vi "Inverse_Kinematics.vi"(4 "arm2 length (mm)":dbl, 6 "arm1 length (mm)":dbl, 9 "arm direction":bool, 10 "y (mm)":dbl, 11 "x (mm)":dbl) -> (2 "th2":dbl, 3 "th1":dbl)   [LabVIEW 2017, in "myPAM.lvlib"]
uses:
  myPAM.lvlib
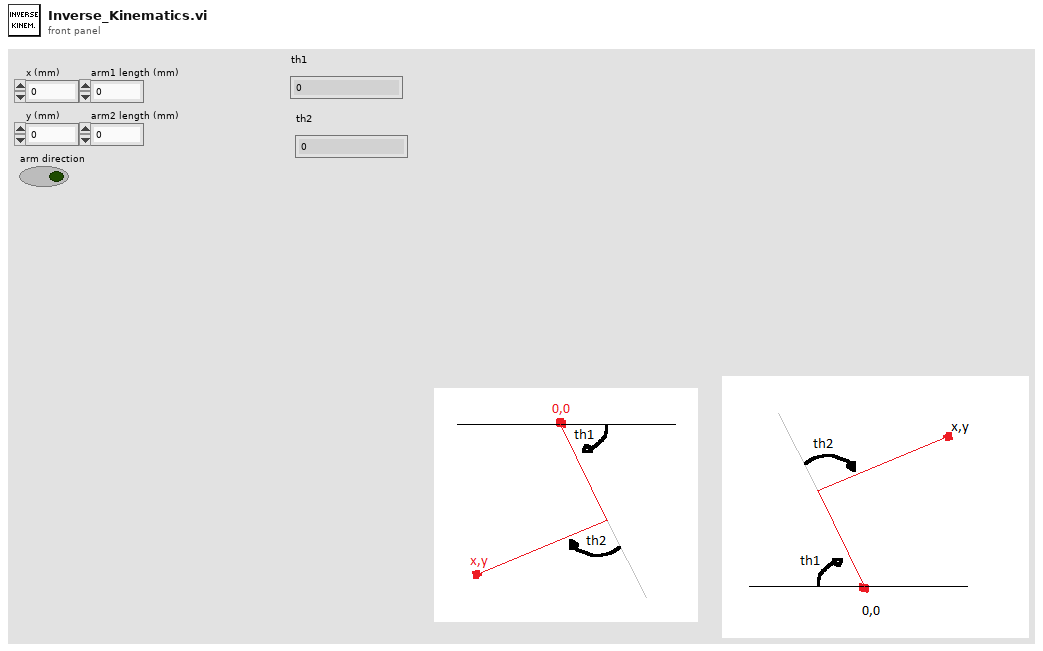
[diagram p1: front panel]
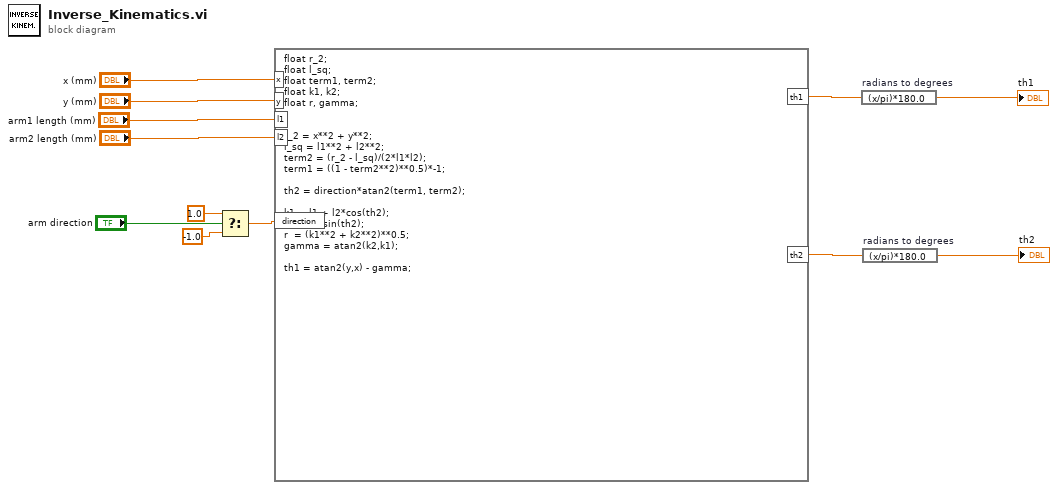
[diagram p0: block diagram]
diagram:
  n1 = Select(t=1.0, s="arm direction", f=-1.0 ("t")) -> (s? t:f=w1:dbl)
  n2 = formula code="float r_2;\nfloat l_sq;\nfloat term1, term2;\nfloat k1, k2;\nfloat r, gamma;\n\n\nr_2 = x**2 + y**2;\nl_sq = l1**2 + l2**2;\nterm2 = (r_2 - l_sq)/(2*l1*l2);\nterm1 = ((1 - term2**2)**0.5)*-1;\n\nth2 = direction*atan2(term1, term2);\n\nk1 = l1 + l2*cos(th2);\nk2 = l2*sin(th2);\nr  = (k1**2 + k2**2)**0.5;\ngamma = atan2(k2,k1);\n\nth1 = atan2(y,x) - gamma;"("x"="x (mm)", "y"="y (mm)", "l1"="arm1 length (mm)", "l2"="arm2 length (mm)", "direction"=w1) -> ("th1"=w4:dbl, "th2"=w5:dbl)
  n3 = expression code="(x/pi)*180.0" "radians to degrees"(w4) -> (→"th1":dbl)
  n4 = expression code="(x/pi)*180.0" "radians to degrees"(w5) -> (→"th2":dbl)
